vi "LogDBCloseRef.vi"(8 "error in (no error)":errorcluster, 10 "enable":bool, 11 "Refnum in":T1) -> (0 "error out":errorcluster, 3 "Refnum out":T1)   [LabVIEW 2011]
uses:
  <vilib>/addons/database/Connection.llb/Conn ObjectReference.ctl
  <vilib>/addons/database/NI_Database_API.lvlib
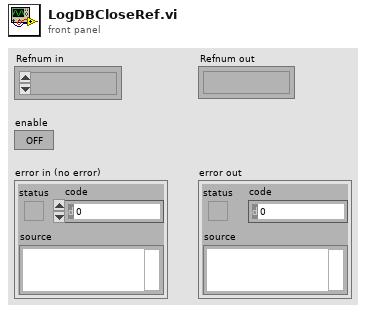
[diagram p1: front panel]
types:
  T1 = typedef "NI_Database_API.lvlib/Conn ObjectReference.ctl" = refnum<k1>
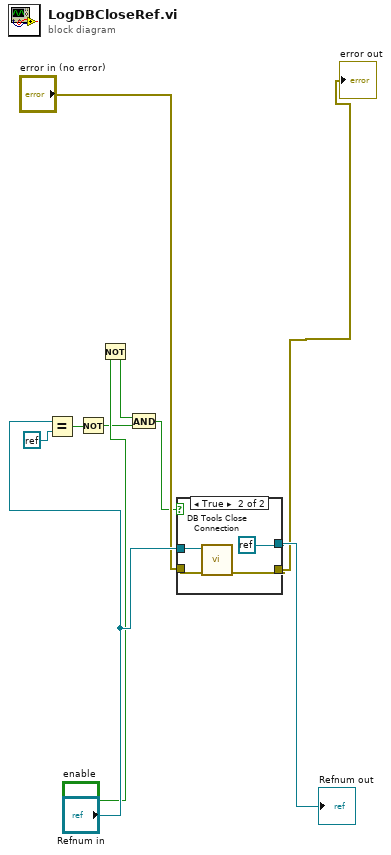
[diagram p0: block diagram]
diagram:
  n1 = Equal?(x="Refnum in", y=refnum<k0> refnum) -> (x = y?=w2:bool)
  n2 = Not(x=w2) -> (.not. x?=w4:bool)
  n3 = Not(x="enable") -> (.not. x?=w3:bool)
  n4 = And(x=w3, y=w4) -> (x .and. y?=w6:bool)
  n5 = case shown="True" w6 {
    tunnel: [w12 w16] -> w1
    tunnel: [w11 refnum<k0> refnum] -> w7
    tunnel: "error in (no error)" -> [w12 w14]
    tunnel: "Refnum in" -> [w11 w13]
    frame False {
    }
    frame True {
      n6 = call <vilib>:"DB Tools Close Connection.vi"("error in (no error)"=w14, "connection reference"=w13) -> ("error out"=w16:errorcluster)  [unwired: 5 in]
    }
  }
  "error out" <- w1
  "Refnum out" <- w7
